vi "Tone Pattern Test.vi"() -> ()   [LabVIEW 2020]
uses:
  Waveform VIs/Tone Pattern VIs/TonePattern-Properties.ctl
  Waveform VIs/Tone Pattern VIs/TonePattern-Data.ctl
panel:
  in  "Save Button":bool
  out "exit signal":bool
  out "Graph":dbl[](graph)
  out "finished":errorcluster
  out "Y-axis":dbl(slide) scale=0.0..3.338035084978648
  in  "Play Button":bool
  in  "Refresh Button":bool
  in  "Quit Button":bool
  out "Mask":i32[][](graph)
  in  "Frame size (s)":dbl=0.25
  in  "Sampling rate (Hz)":dbl=50000.0
  in  "Properties":T1={"Freq"={"Min (Hz)"=222.0, "Max (Hz)"=2000.0, "#/octave"=6}, "Time"={"Duration (ms)"=50.0, "Interval (ms)"=50.0, "Ramp (ms)"=5.0}, "Pattern"={"# rand"=2.0, "reg fraction"=1.0, "Rcyc"=10, "pattern"=enum."RAND-REG", "Lsignal (cyc)"={"Min"=7, "Max"=9}, "Trans (cyc)"={"Min"=4, "Max"=5}}}
  in  "Stop Button":bool
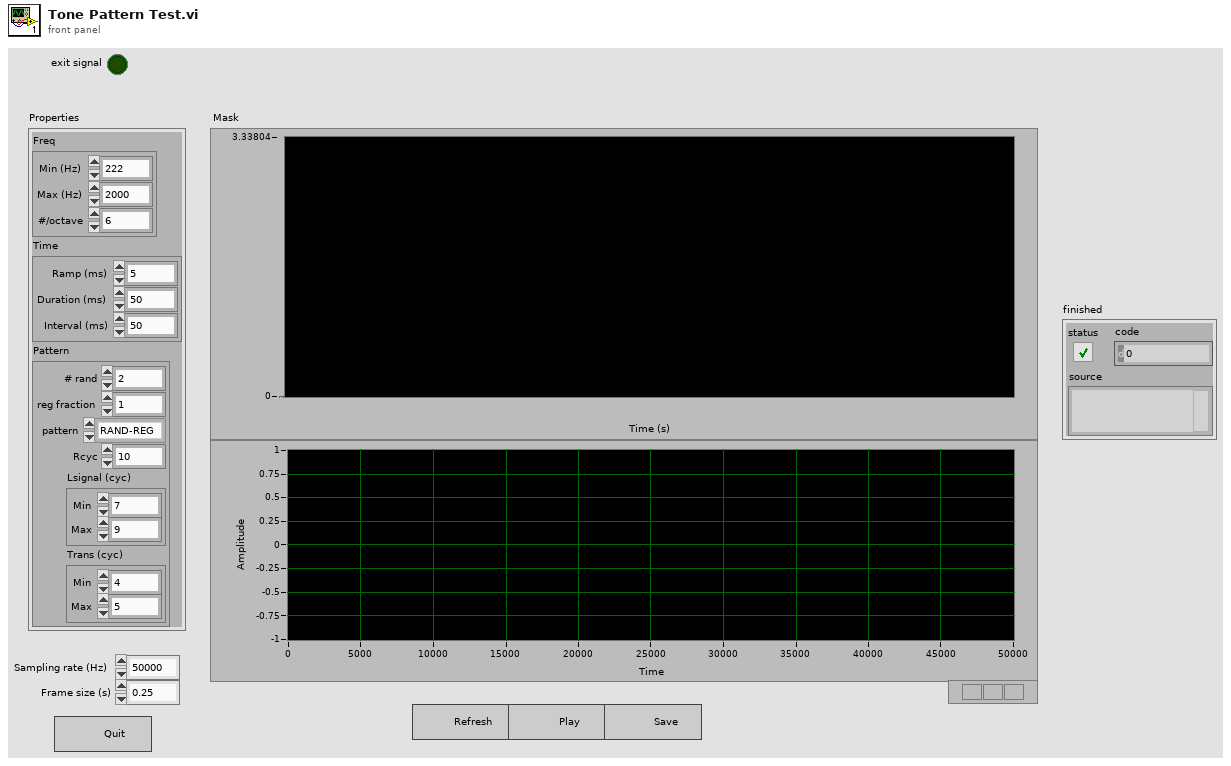
[diagram p1: front panel]
types:
  T1 = typedef "TonePattern-Properties.ctl" = cluster{"Freq":cluster{"Min (Hz)":dbl, "Max (Hz)":dbl, "#/octave":i32}, "Time":cluster{"Duration (ms)":dbl, "Interval (ms)":dbl, "Ramp (ms)":dbl}, "Pattern":cluster{"# rand":dbl, "reg fraction":dbl, "Rcyc":i32, "pattern":enum16{"RAND-REG", "REG-RAND", "RAND", "REG", "STEP", "CF"}, "Lsignal (cyc)":cluster{"Min":i32, "Max":i32}, "Trans (cyc)":cluster{"Min":i32, "Max":i32}}}
  T2 = typedef "TonePattern-Data.ctl" = cluster{"Tones":dbl[][], "Mask":i32[], "Index":i32, "pts/clock":i32, "leftover":i32, "pts/tone":i32, "transition":i32, "nrepeat":i32}
  T3 = enum8{"Enabled", "Disabled", "Disabled and Grayed Out"}
  T4 = cluster{"Data":T2, "Sampling rate (Hz)":dbl, i32, "#frames":i32}
  T5 = typedef "Sound Output Task ID.ctl" = u32
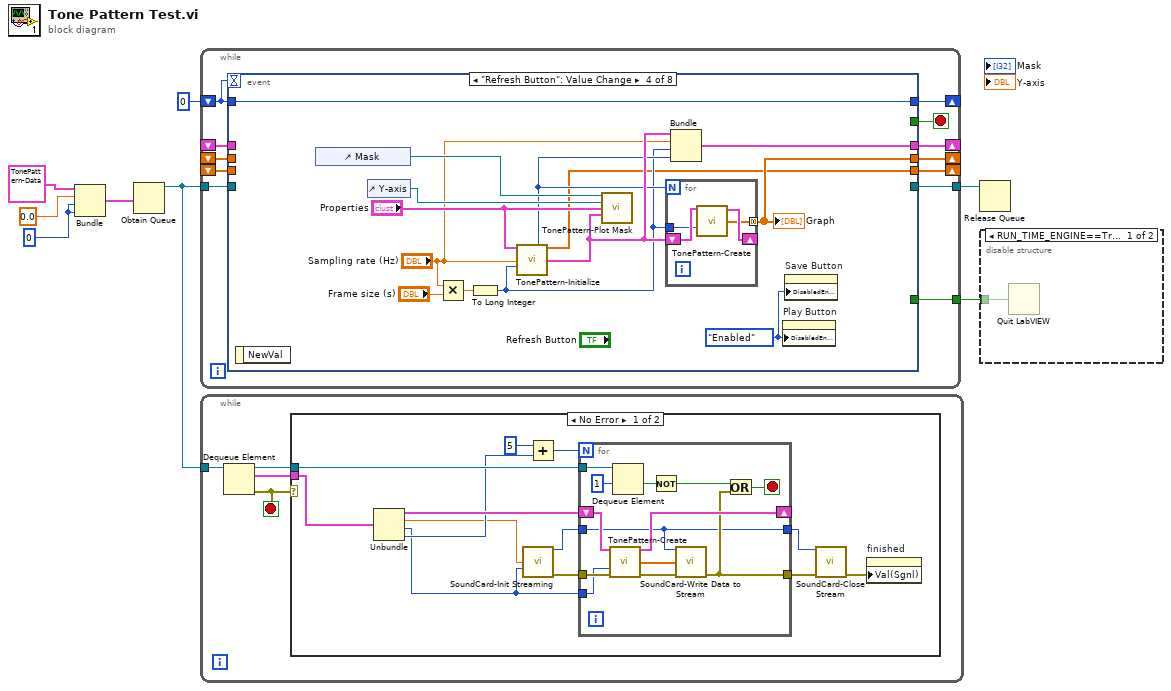
[diagram p0: block diagram]
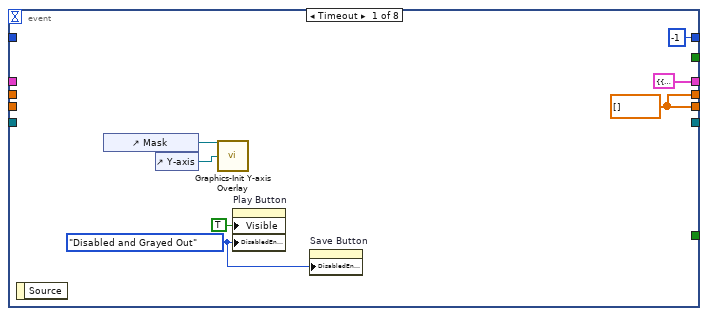
[diagram p4: hidden frame]
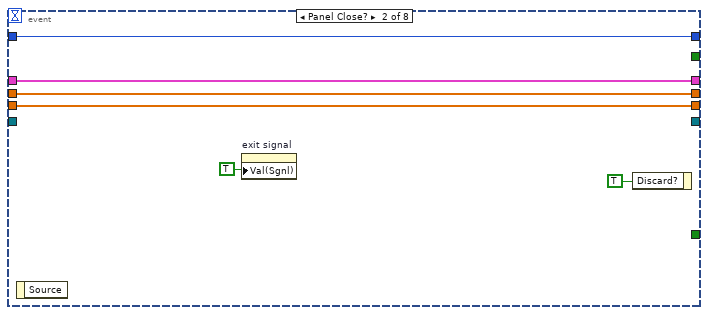
[diagram p5: hidden frame]
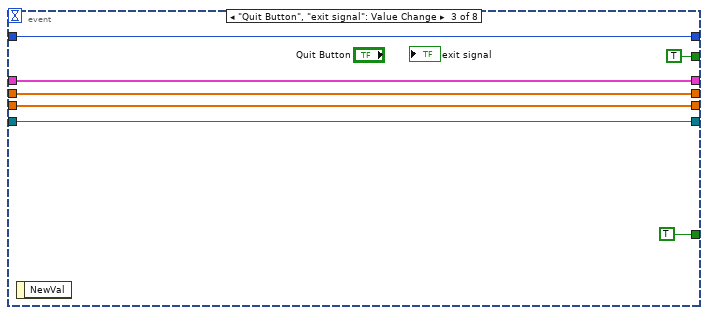
[diagram p6: hidden frame]
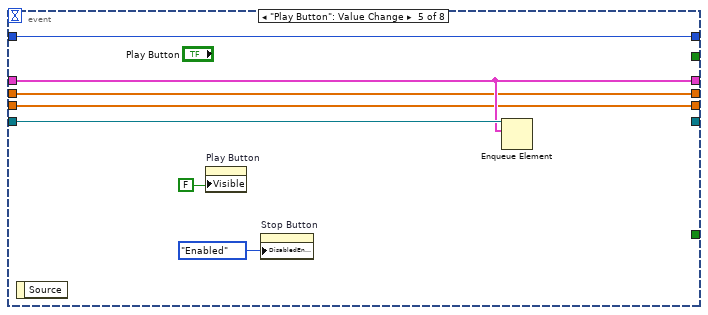
[diagram p7: hidden frame]
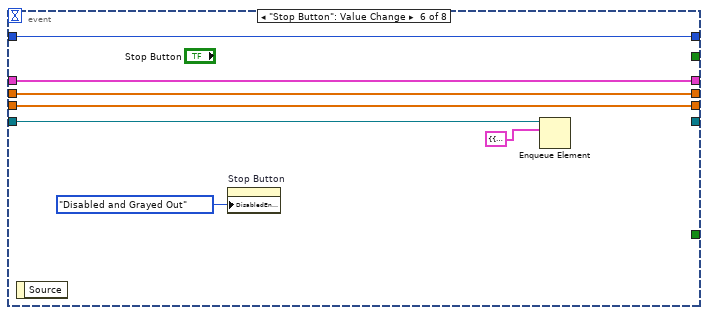
[diagram p8: hidden frame]
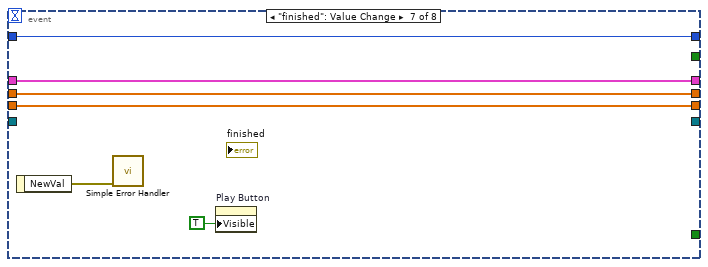
[diagram p9: hidden frame]
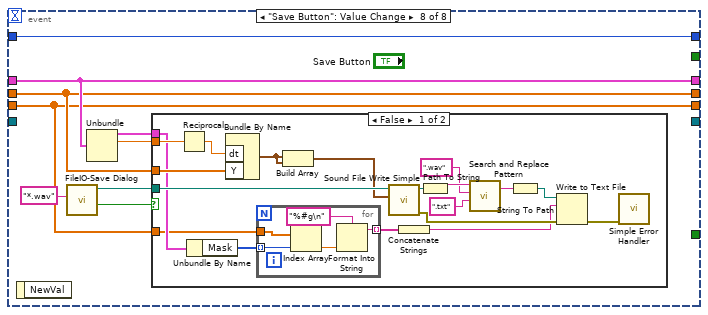
[diagram p10: hidden frame]
diagram:
  w2 = 0
  n1 = Bundle("Data"=T2 {"Tones"=array17x5000[85000 elements], "Mask"=[8], "Index"=0, "pts/clock"=5000, "leftover"=0, "pts/tone"=5000, "transition"=0, "nrepeat"=0}, 0.0, w2, w2) -> (w5:cluster{"Data":T2, dbl, i32, i32})  [unwired: 1 in]
  n2 = Obtain Queue(element data type=w5) -> (queue out=w6:refnum<queue>)  [unwired: 4 in, 2 out]
  n3 = while {
    shift-right: [w18] -> _
    shift-left: 0 -> [w19]
    tunnel: w6 -> [w17]
    tunnel: [w16] -> w7
    tunnel: [w15] -> w1
    shift-right: [w14] -> _
    shift-left: _ -> [w13]
    shift-right: [w12] -> _
    shift-left: _ -> [w11]
    shift-right: [w10] -> _
    shift-left: _ -> [w9]
    stop <- w20 stop-if-true
    n4 = event shown="[3] \"Refresh Button\": Value Change" {
      selector: _ -> [_ _ _ _ _ _ _ _]
      dyn-events: _ -> [_ _ _ _ _ _ _ _]
      timeout: w19 -> [_ _ _ _ _ _ _ _]
      tunnel: [_ _ TRUE _ _ _ _ _] -> w20
      tunnel: w19 -> [_ w33 w39 w53 w65 w72 w78 w87]
      tunnel: [-1 w33 w39 w53 w65 w72 w78 w87] -> w18
      tunnel: w17 -> [_ _ w38 _ w62 w71 _ _]
      tunnel: [_ _ w38 _ _ _ _ _] -> w16
      tunnel: [_ _ TRUE _ _ _ _ _] -> w15
      tunnel: [cluster{"Data":T2, dbl, i32, i32} {"Data"={"Tones"=[], "Mask"=[], "Index"=0, "pts/clock"=0, "leftover"=0, "pts/tone"=0, "transition"=0, "nrepeat"=0}, 0.0, 0, 0} ("output cluster") w30 w36 w44 w61 w68 w75 w83] -> w14
      tunnel: w13 -> [_ w30 w36 _ w61 w68 w75 w83]
      tunnel: [w21 w29 w35 w43 w60 w67 w74 w81] -> w12
      tunnel: w11 -> [_ w29 w35 _ w60 w67 w74 w81]
      tunnel: [w21 w28 w34 w41 w59 w66 w73 w79] -> w10
      tunnel: w9 -> [_ w28 w34 _ w59 w66 w73 w79]
      event Timeout {
        w21 = dbl[] [] ("Y")
        w22 = T3."Disabled and Grayed Out" ("Disabled")
        n5 = event-data() -> ()  [unwired: 1 in, 1 out]
        n6 = control-ref of="Mask"() -> (w26:refnum<vi>)
        n7 = control-ref of="Y-axis"() -> (w27:refnum<vi>)
        n8 = call "Graphics-Init Y-axis Overlay.vi"("Ctl Refnum"=w26, "Y-axis slider"=w27) -> ()  [unwired: 13 in, 1 out]
        n9 = property on="Play Button" class="Bool"("Visible"=TRUE, "DisabledEnum"=w22) -> ()  [unwired: 2 in, 2 out]
        n10 = property on="Save Button" class="Bool"("DisabledEnum"=w22) -> ()  [unwired: 2 in, 2 out]
      }
      event Panel Close? {
        n11 = event-data() -> ()  [unwired: 1 in, 1 out]
        n12 = property on="exit signal" class="Bool (strict)"("Val(Sgnl)"=TRUE ("Value (Signaling)")) -> ()  [unwired: 2 in, 2 out]
        n13 = event-data("Discard?"=TRUE) -> ()  [unwired: 1 in, 1 out]
      }
      event "Quit Button", "exit signal": Value Change {
        n14 = event-data() -> ()  [unwired: 1 in, 1 out]
      }
      event "Refresh Button": Value Change {
        w42 = T3."Enabled" ("Disabled")
        n15 = event-data() -> ()  [unwired: 1 in, 1 out]
        n16 = control-ref of="Mask"() -> (w54:refnum<vi>)
        n17 = control-ref of="Y-axis"() -> (w52:refnum<vi>)
        n18 = Multiply(x="Sampling rate (Hz)", y="Frame size (s)") -> (x*y=w51:dbl)
        n19 = To Long Integer(number=w51) -> (32bit integer=w45:i32)
        n20 = call "TonePattern-Initialize.vi"("Tone Cloud"="Properties", "Sampling rate (Hz)"="Sampling rate (Hz)", "Npts"=w45) -> ("#frames"=w46:i32, "Freqs"=w41:dbl[], "Data"=w48:T2)  [unwired: 9 in, 1 out]
        n21 = call "TonePattern-Plot Mask.vi"("Graph"=w54, "Y-axis slider"=w52, "Properties"="Properties", "Data"=w48) -> ()  [unwired: 11 in, 1 out]
        n22 = for {
          N: w46 -> [_]
          tunnel: w45 -> [w55]
          shift-right: [w57] -> _
          shift-left: w48 -> [w58]
          tunnel: [w56] -> w43 mode=concatenating
          n23 = call "TonePattern-Create.vi"("Data in"=w58, "Npts"=w55) -> ("Data out"=w57:T2, "Y"=w56:dbl[])  [unwired: 11 in, 1 out]
        }
        "Graph" <- w43
        n24 = Bundle("Data"=w48, "Sampling rate (Hz)"="Sampling rate (Hz)", w45, "#frames"=w46) -> (w44:T4)  [unwired: 1 in]
        n25 = property on="Play Button" class="Bool"("DisabledEnum"=w42) -> ()  [unwired: 2 in, 2 out]
        n26 = property on="Save Button" class="Bool"("DisabledEnum"=w42) -> ()  [unwired: 2 in, 2 out]
      }
      event "Play Button": Value Change {
        n27 = event-data() -> ()  [unwired: 1 in, 1 out]
        n28 = property on="Play Button" class="Bool"("Visible"=FALSE) -> ()  [unwired: 2 in, 2 out]
        n29 = property on="Stop Button" class="Bool"("DisabledEnum"=T3."Enabled" ("Disabled")) -> ()  [unwired: 2 in, 2 out]
        n30 = Enqueue Element(queue=w62, element=w61) -> ()  [unwired: 2 in, 3 out]
      }
      event "Stop Button": Value Change {
        n31 = event-data() -> ()  [unwired: 1 in, 1 out]
        n32 = property on="Stop Button" class="Bool"("DisabledEnum"=T3."Disabled and Grayed Out" ("Disabled")) -> ()  [unwired: 2 in, 2 out]
        n33 = Enqueue Element(queue=w71, element=cluster{"Data":T2, dbl, i32, i32} {"Data"={"Tones"=[], "Mask"=[], "Index"=0, "pts/clock"=0, "leftover"=0, "pts/tone"=0, "transition"=0, "nrepeat"=0}, 0.0, 0, 0}) -> ()  [unwired: 2 in, 3 out]
      }
      event "finished": Value Change {
        n34 = event-data() -> ("NewVal"=w77:errorcluster)  [unwired: 1 in]
        n35 = call <vilib>:"Simple Error Handler.vi"("error in (no error)"=w77) -> ()  [unwired: 4 in, 5 out]
        n36 = property on="Play Button" class="Bool"("Visible"=TRUE) -> ()  [unwired: 2 in, 2 out]
      }
      event "Save Button": Value Change {
        n37 = event-data() -> ()  [unwired: 1 in, 1 out]
        n38 = call "FileIO-Save Dialog.vi"("pattern (all files)"="*.wav") -> ("cancelled"=w85:bool, "selected path"=w84:path)  [unwired: 8 in, 1 out]
        n39 = Unbundle(w83) -> ("Data"=w80:T2, "Sampling rate (Hz)"=w82:dbl)  [unwired: 2 out]
        n40 = case shown="False" w85 {
          tunnel: w84 -> [w106 _]
          tunnel: w82 -> [w105 _]
          tunnel: w81 -> [w103 _]
          tunnel: w80 -> [w100 _]
          tunnel: w79 -> [w98 _]
          frame False {
            n41 = Reciprocal(x=w105) -> (1/x=w104:dbl)
            n42 = Unbundle By Name(w100) -> ("Mask"=w99:i32[])
            n43 = Bundle By Name("dt"=w104, "Y"=w103) -> (w101:waveform(dbl))  [unwired: 1 in]
            n44 = for {
              tunnel: w99 -> [w110] mode=indexing
              tunnel: w98 -> [w111]
              tunnel: [w108] -> w89 mode=indexing
              n45 = Index Array(array=w111, index=w110) -> (element=w109:dbl)
              n46 = Format Into String(format string="%#g\n", w109) -> (resulting string=w108:string)  [unwired: 2 in, 1 out]
            }
            n47 = Build Array(w101, w101) -> (w102:waveform(dbl)[])
            n48 = call <vilib>:"Sound File Write Simple.vi"("data"=w102, "path"=w106) -> ("error out"=w92:errorcluster, "path out"=w97:path)  [unwired: 8 in]
            n49 = Concatenate Strings(w89) -> (w88:string)
            n50 = Path To String(path=w97) -> (string=w96:string)
            n51 = call <vilib>:"Search and Replace Pattern.vi"("string"=w96, "regular expression (\"\")"=".wav" ("regular expression (\"\")"), "replace string (\"\")"=".txt" ("replace string (\"\")")) -> ("result string"=w93:string)  [unwired: 2 in, 1 out]
            n52 = String To Path(string=w93) -> (path=w91:path)
            n53 = Write to Text File(file (use dialog)=w91, text=w88, error in=w92) -> (error out=w90:errorcluster)  [unwired: 1 in, 2 out]
            n54 = call <vilib>:"Simple Error Handler.vi"("error in (no error)"=w90) -> ()  [unwired: 4 in, 5 out]
          }
          frame True {
          }
        }
      }
    }
  }
  n55 = while {
    tunnel: w6 -> [w115]
    stop <- w112 stop-if-true
    n56 = Dequeue Element(queue=w115) -> (queue out=w113:refnum<queue>, element=w114:cluster{"Data":T2, dbl, i32, i32}, error out=w112:errorcluster)  [unwired: 2 in, 1 out]
    n57 = case shown="No Error" w112 {
      tunnel: w114 -> [w120 _]
      tunnel: w113 -> [w128 _]
      frame No Error {
        n58 = Unbundle(w120) -> ("Data"=w119:T2, w116:dbl, w117:i32, w118:i32)
        n59 = call "SoundCard-Init Streaming.vi"("sample rate (S/s)"=w116, "Npts"=w117) -> ("task ID"=w126:T5, "error out"=w127:errorcluster)  [unwired: 12 in]
        n60 = Add(x=5, y=w118) -> (x+y=w122:i32)
        n61 = for {
          N: w122 -> [_]
          tunnel: w128 -> [w141]
          tunnel: w127 -> [w136]
          tunnel: [w132] -> w125
          shift-right: [w134] -> _
          shift-left: w119 -> [w135]
          tunnel: w117 -> [w129]
          tunnel: w126 -> [w131]
          tunnel: [w131] -> w123
          stop <- w137 stop-if-true
          n62 = call "TonePattern-Create.vi"("Data in"=w135, "Npts"=w129, "error in (no error)"=w136) -> ("Data out"=w134:T2, "Y"=w130:dbl[], "error out"=w133:errorcluster)  [unwired: 10 in]
          n63 = Dequeue Element(queue=w141, timeout in ms (-1)=1) -> (timed out?=w139:bool)  [unwired: 1 in, 3 out]
          n64 = Not(x=w139) -> (.not. x?=w138:bool)
          n65 = call "SoundCard-Write Data to Stream.vi"("task ID"=w131, "Array"=w130, "error in (no error)"=w133) -> ("error out"=w132:errorcluster)  [unwired: 11 in, 1 out]
          n66 = Or(x=w138, y=w132) -> (x .or. y?=w137:bool)
        }
        n67 = call "SoundCard-Close Stream.vi"("task ID"=w123, "error in (no error)"=w125) -> ("error out"=w124:errorcluster)  [unwired: 13 in]
        n68 = property on="finished" class="Clust (strict)"("Val(Sgnl)"=w124) -> ()  [unwired: 2 in, 2 out]
      }
      frame Error {
      }
    }
  }
  n69 = Release Queue(queue=w7) -> ()  [unwired: 2 in, 3 out]
  n70 = disable-structure shown="RUN_TIME_ENGINE==True" {
    disable-tunnel: w1 -> [w142 _]
    frame condition #0 {
      n71 = Quit LabVIEW(quit? (T)=w142) -> ()
    }
    frame condition #1 (active) {
    }
  }
